vi "8bit sync-Gen patches montage.vi"(0 "U8 Image (Montage)":T2, 2 "AVI Refnum in":T3, 3 "Image Array(Single Trial)":u8[][][](array[numeric]), 5 "error in (no error)":errorcluster, 6 "Coordinates of montage positions":cluster{"X\n\nY":i32[]}[](array[cluster]), 8 "Patch frame index":i32, 9 "Frames info":T4, 10 "Number of Frames in a Cycle":i32, 11 "Image refs cluster":T1) -> (14 "AVI Refnum out":T3, 16 "U8 Image (Montage)":T2, 19 "error out":errorcluster)   [LabVIEW 2017]
uses:
  <vilib>/vision/Image Controls.llb/IMAQ Image.ctl
  <vilib>/vision/Avi.llb/IMAQ AVI2 Refnum.ctl
  Typedefs/8bit sync-IMAQ image refs.ctl
  Globals/gl_8-bit montage window ctrl refs.vi
  <vilib>/vision/NI_Vision_Development_Module.lvlib
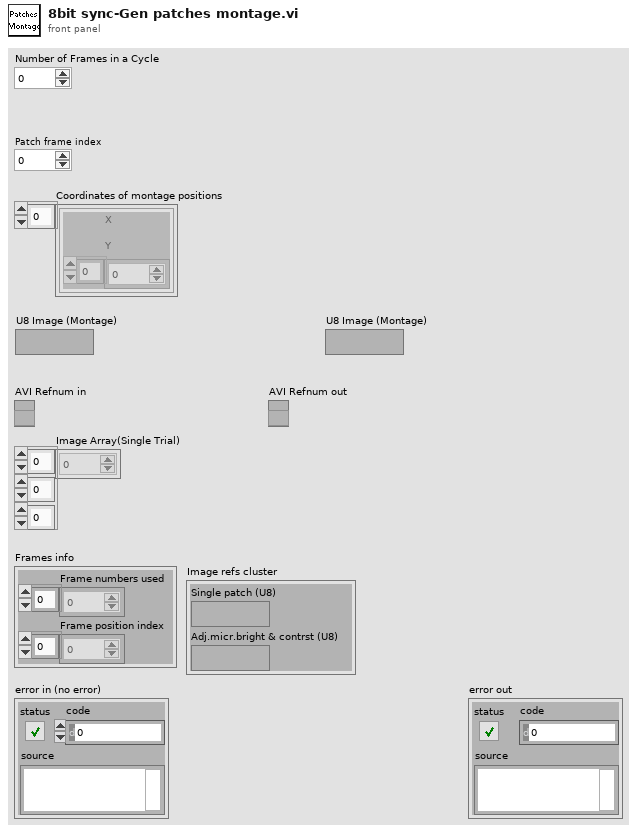
[diagram p1: front panel]
types:
  T1 = typedef "8bit sync-IMAQ image refs.ctl" = cluster{"Single patch (U8)":T2, "Adj.micr.bright & contrst (U8)":T2}
  T2 = typedef "IMAQ Image.ctl" = refnum<image>
  T3 = typedef "IMAQ AVI2 Refnum.ctl" = refnum<k20>
  T4 = cluster{"Frame numbers used":i32[], "Frame position index":i32[]}
  T5 = typedef "8-bit video export window ctrl refs.ctl" = cluster{"This VI":refnum<vi>, "Add speed data":refnum<vi>, "Add camera videos":refnum<vi>, "Stop button":refnum<vi>, "Camera Video Adjustments":refnum<vi>, "Microscope Image Adjustments":refnum<vi>, "Execute":refnum<vi>, "Codec":refnum<vi>, "Channel to load":refnum<vi>, "Speed graph behaviour":refnum<vi>, "Include speed graph":refnum<vi>, "Number of rows to generate":refnum<vi>, "Path":refnum<vi>}
  T6 = typedef "Bright-Contr-Gamma cluster.ctl" = cluster{"Brightness":sgl, "Contrast":sgl, "Gamma":sgl}
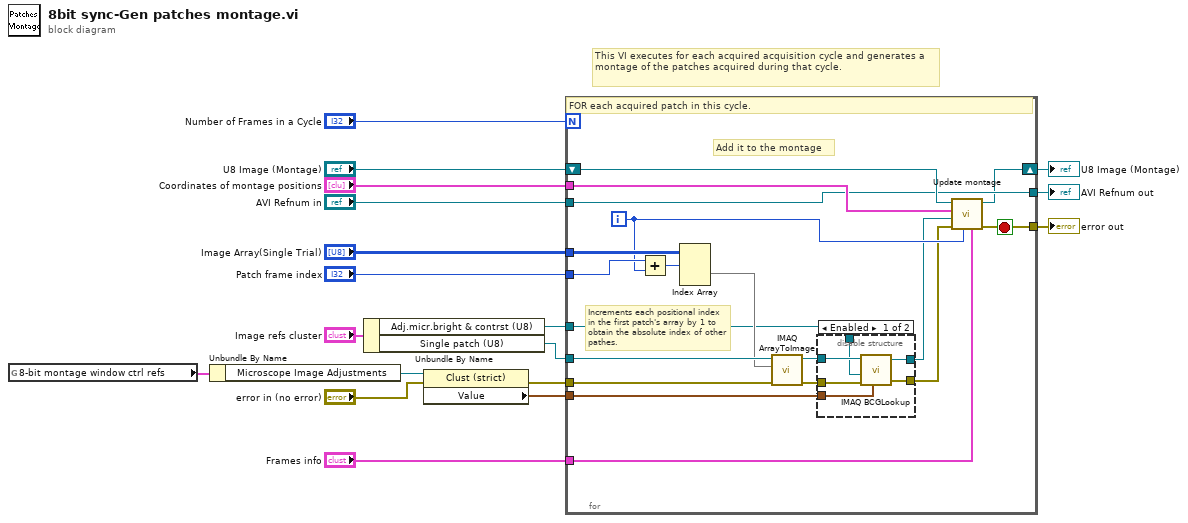
[diagram p0: block diagram]
diagram:
  # "This VI executes for each acquired acquisition cycle and generates a montage of the patches acquired during that cycle."
  n1 = global read "gl_8-bit montage window ctrl refs.vi" "8-bit montage window ctrl refs"() -> (w6:T5)
  n2 = Unbundle By Name(w6) -> ("Microscope Image Adjustments"=w7:refnum<vi>)
  n3 = Unbundle By Name("Image refs cluster") -> ("Adj.micr.bright & contrst (U8)"=w2:T2, "Single patch (U8)"=w8:T2)
  n4 = property class="Clust (strict)"(reference=w7, error in="error in (no error)") -> (error out=w3:errorcluster, "Value"=w4:T6)  [unwired: 1 out]
  n5 = for {
    N: "Number of Frames in a Cycle" -> [_]
    tunnel: "Image Array(Single Trial)" -> [w37]
    tunnel: "AVI Refnum in" -> [w28]
    tunnel: [w26] -> w17
    tunnel: w8 -> [w36]
    tunnel: [w28] -> w15
    tunnel: w3 -> [w34]
    shift-right: [w27] -> w16
    shift-left: "U8 Image (Montage)" -> [w33]
    tunnel: "Coordinates of montage positions" -> [w32]
    tunnel: "Frames info" -> [w29]
    tunnel: "Patch frame index" -> [w31]
    tunnel: w4 -> [w21]
    tunnel: w2 -> [w19]
    i -> [w30]
    stop <- w26 stop-if-true
    # "Add it to the montage"
    # "Increments each positional index in the first patch's array by 1 to obtain the absolute index of other pathes."
    # "FOR each acquired patch in this cycle."
    n6 = Add(x=w31, y=w30) -> (x+y=w35:i32)
    n7 = Index Array(array=w37, index (dim 0)=w35) -> (element=w25:u8[][])  [unwired: 2 in]
    n8 = call "IMAQ ArrayToImage"("error in (no error)"=w34, "Image Pixels (U8)"=w25, "Image"=w36) -> ("error out"=w22:errorcluster, "Image Out"=w20:T2)  [unwired: 7 in]
    n9 = disable-structure shown="Enabled" {
      disable-tunnel: [w43 w45] -> w24
      disable-tunnel: [w42 w44] -> w23
      disable-tunnel: w22 -> [w41 w44]
      disable-tunnel: w21 -> [w38 _]
      disable-tunnel: w20 -> [w40 w45]
      disable-tunnel: w19 -> [w39 _]
      frame Enabled {
        n10 = call "IMAQ BCGLookup"("Image Src"=w40, "BCG Values"=w38, "Image Dst"=w39, "error in (no error)"=w41) -> ("Image Dst Out"=w43:T2, "error out"=w42:errorcluster)  [unwired: 3 in]
      }
      frame Disabled {
      }
    }
    n11 = call "Update montage.vi"("Frames info"=w29, "Frame's rel. index"=w30, "Error in"=w23, "Single patch image"=w24, "Coordinates of montage positions"=w32, "Image (Montage)"=w33) -> ("error out"=w26:errorcluster, "Image (Montage)"=w27:T2)  [unwired: 4 in]
  }
  "error out" <- w17
  "U8 Image (Montage)" <- w16
  "AVI Refnum out" <- w15
